vi "testGetConfig.vi"(8 "error in (no error)":errorcluster) -> (0 "error out":errorcluster)   [LabVIEW 2018]
uses:
  <vilib>/addons/_JKI Toolkits/Caraya/classes/Assert/Assert Equal Value and Type_Variant.vi
  <vilib>/addons/_JKI Toolkits/Caraya/classes/Test/Test.lvclass
  <vilib>/addons/_JKI Toolkits/Caraya/classes/Assert/Assert.lvclass
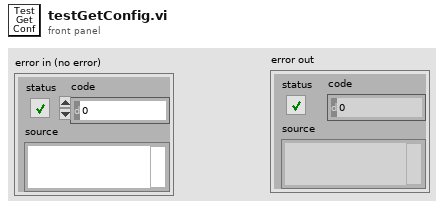
[diagram p1: front panel]
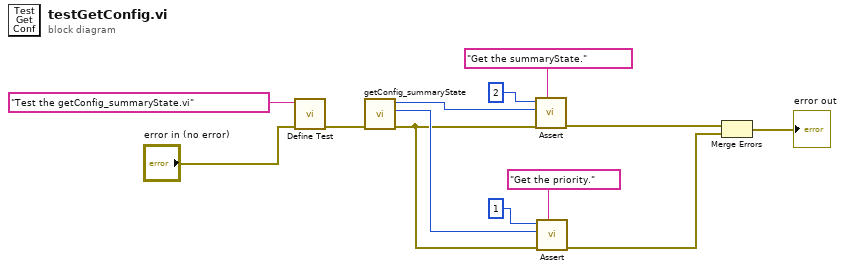
[diagram p0: block diagram]
diagram:
  n1 = call <vilib>:"Define Test.vi"("error in (no error)"="error in (no error)", "Label (VI Title)"="Test the getConfig_summaryState.vi") -> ("error out"=w11:errorcluster)  [unwired: 9 in]
  n2 = call "getConfig_summaryState.vi"("error in (no error)"=w11) -> ("error out"=w7:errorcluster, "priority"=w8:i32, "summaryState"=w10:i32)  [unwired: 8 in]
  n3 = call-poly <vilib>:"Assert.vi"("Label"="Get the summaryState.", "error in (no error)"=w7, "Y"=w10, "X"=2) -> ("error out"=w5:errorcluster)  [unwired: 7 in]
  n4 = call-poly <vilib>:"Assert.vi"("Label"="Get the priority.", "error in (no error)"=w7, "Y"=w8, "X"=1) -> ("error out"=w4:errorcluster)  [unwired: 7 in]
  n5 = Merge Errors(w5, w4) -> (→"error out":errorcluster)
